vi "test Convert Endpoint to UI Element.vi"(8 "error in (no error)":errorcluster, 11 "TestCase in":refnum<class "NI-SWITCH Unit Tests.lvclass">) -> (0 "error out":errorcluster, 3 "TestCase out":refnum<class "NI-SWITCH Unit Tests.lvclass">)   [LabVIEW 2017, in "NI-SWITCH Unit Tests.lvclass"]
uses:
  NI-SWITCH Unit Tests.lvclass
  Shared/Endpoint Configuration Enum.ctl
  System Explorer/Channel Type.ctl
  Shared/Endpoint Configuration Cluster.ctl
  <vilib>/addons/_JKI Toolkits/VI Tester/TestCase.llb/TestCase.lvclass
  System Explorer/NI-SWITCH System Explorer.lvlib
  Shared/NI-SWITCH Shared.lvlib
  C:/Program Files (x86)/National Instruments/LabVIEW 2017/vi.lib/addons/_JKI Toolkits/VI Tester/TestCase.llb/TestCase.lvclass
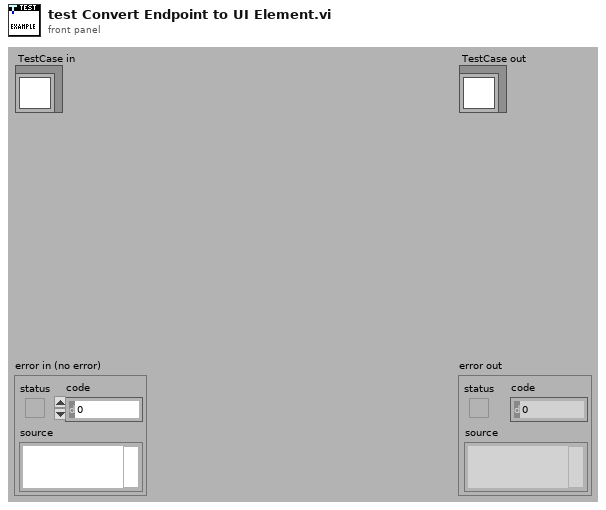
[diagram p1: front panel]
types:
  T1 = typedef "NI-SWITCH Shared.lvlib/Endpoint Configuration Enum.ctl" = enum16{"Load", "Source", "Configuration"}
  T2 = typedef "NI-SWITCH System Explorer.lvlib/Channel Type.ctl" = enum16{"Load (Default)", "Source", "Configuration"}
  T3 = cluster{"Configuration":T1, "Configuration 2":T2}[]
  T4 = typedef "NI-SWITCH Shared.lvlib/Endpoint Configuration Cluster.ctl" = cluster{"Endpoint":string, "Configuration":T1}
  T5 = typedef "NI-SWITCH System Explorer.lvlib/Channel.ctl" = cluster{"Endpoint":string, "Configuration":T2}
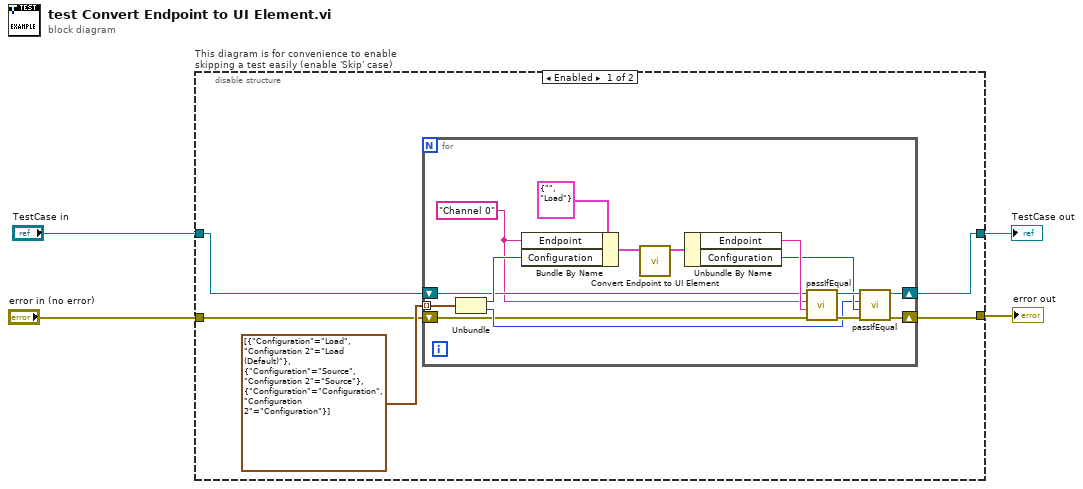
[diagram p0: block diagram]
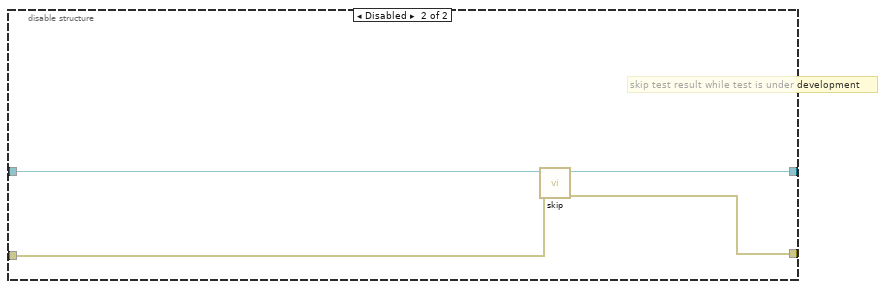
[diagram p2: hidden frame]
diagram:
  n1 = disable-structure "This diagram is for convenience to enable skipping a test easily (enable 'Skip' case)" shown="Enabled" {
    disable-tunnel: "TestCase in" -> [w6 w28]
    disable-tunnel: [w5 w26] -> w1
    disable-tunnel: [w7 w27] -> w3
    disable-tunnel: "error in (no error)" -> [w8 w25]
    frame Enabled {
      n2 = for {
        tunnel: T3 [{"Configuration"=enum."Load", "Configuration 2"=enum."Load (Default)"}, {"Configuration"=enum."Source", "Configuration 2"=enum."Source"}, {"Configuration"=enum."Configuration", "Configuration 2"=enum."Configuration"}] -> [w18] mode=indexing
        shift-right: [w14] -> w7
        shift-left: w8 -> [w15]
        shift-right: [w12] -> w5
        shift-left: w6 -> [w13]
        w10 = "Channel 0" ("Endpoint")
        n3 = Unbundle(w18) -> ("Configuration"=w17:T1, "Configuration 2"=w16:T2)
        n4 = Bundle By Name(cluster=T4 {"Endpoint"="", "Configuration"=enum."Load"} ("Connection"), "Endpoint"=w10, "Configuration"=w17) -> (w11:T4)
        n5 = call "Convert Endpoint to UI Element.vi"("Connection"=w11) -> ("Channel"=w24:T5)  [unwired: 10 in]
        n6 = Unbundle By Name(w24) -> ("Endpoint"=w20:string, "Configuration"=w19:T2)
        n7 = call-dynamic "passIfEqual.vi"("error in (no error)"=w15, "y"=w20, "x"=w10, "TestCase in"=w13) -> ("error out"=w21:errorcluster, "TestCase out"=w22:refnum<class "NI-SWITCH Unit Tests.lvclass">)  [unwired: 6 in]
        n8 = call-dynamic "passIfEqual.vi"("error in (no error)"=w21, "y"=w19, "x"=w16, "TestCase in"=w22) -> ("error out"=w14:errorcluster, "TestCase out"=w12:refnum<class "NI-SWITCH Unit Tests.lvclass">)  [unwired: 6 in]
      }
    }
    frame Disabled {
      # "skip test result while test is under development"
      n9 = call <vilib>:"skip.vi"("error in (no error)"=w25, "TestCase in"=w28) -> ("error out"=w27:errorcluster, "TestCase out"=w26:refnum<class "NI-SWITCH Unit Tests.lvclass">)  [unwired: 8 in]
    }
  }
  "error out" <- w3
  "TestCase out" <- w1
